vi "Highlight Selected Grey.vi"(8 "error in (no error)":errorcluster, 10 "Grey Scale Index (0-255)":u8, 11 "ColorSelector in":refnum<class "ColorSelector.lvclass">) -> (0 "error out":errorcluster, 3 "ColorSelector (dup)":refnum<class "ColorSelector.lvclass">)   [LabVIEW 2015, in "ColorSelector.lvclass"]
doc: "This VI draws the crosshairs on the correct coordinate in the Grey Selector.\n<b> </b> <b> </b>\n©2017 Q Software Innovations, LLC (QSI)\nwritten by Quentin Alldredge\nproduced in LabVIEW 2015\n\nsupport@qsoftwareinnovations.com\nwww.qsoftwareinnovations.com\n\nAll rights reserved.\n\nRedistribution and use in source and binary forms, with or without modification, are permitted provided that the following conditions are met:\n\n * Redistributions of source code must retain the above copyright notice, this list of conditions and the following disclaimer.\n * Redistributions in binary form must reproduce the above copyright notice, this list of conditions and the following disclaimer in the documentation and/or other materials provided with the distribution.\n * Neither the name of Q Software Innovations, LLC. nor the names of its contributors may be used to endorse or promote products derived from this software without specific prior written permission.\n\nTHIS SOFTWARE IS PROVIDED BY THE COPYRIGHT HOLDERS AND CONTRIBUTORS \"AS IS\" AND ANY EXPRESS OR IMPLIED WARRANTIES, INCLUDING, BUT NOT LIMITED TO, THE IMPLIED WARRANTIES OF MERCHANTABILITY AND FITNESS FOR A PARTICULAR PURPOSE ARE DISCLAIMED. IN NO EVENT SHALL THE COPYRIGHT OWNER OR CONTRIBUTORS BE LIABLE FOR ANY DIRECT, INDIRECT, INCIDENTAL, SPECIAL, EXEMPLARY, OR CONSEQUENTIAL DAMAGES (INCLUDING, BUT NOT LIMITED TO, PROCUREMENT OF SUBSTITUTE GOODS OR SERVICES; LOSS OF USE, DATA, OR PROFITS; OR BUSINESS INTERRUPTION) HOWEVER CAUSED AND ON ANY THEORY OF LIABILITY, WHETHER IN CONTRACT, STRICT LIABILITY, OR TORT (INCLUDING NEGLIGENCE OR OTHERWISE) ARISING IN ANY WAY OUT OF THE USE OF THIS SOFTWARE, EVEN IF ADVISED OF THE POSSIBILITY OF SUCH DAMAGE."
uses:
  ColorSelector.lvclass
  ColorSelector.lvclass/ColorSelector.ctl
  Read GreySelectPic.vi
  Read GreyGridCoords.vi
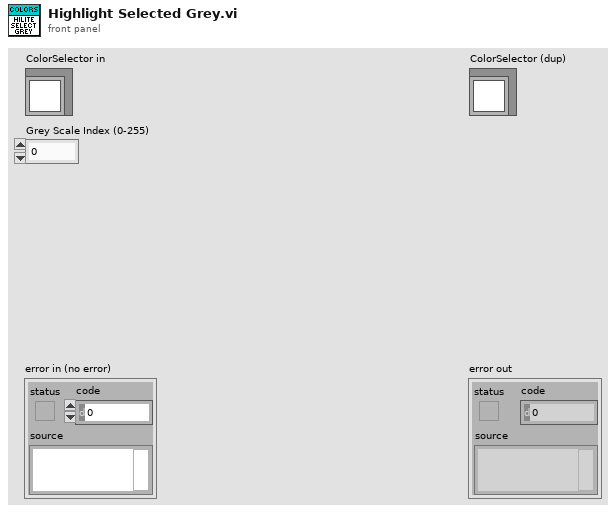
[diagram p1: front panel]
types:
  T1 = cluster{"Width":i16, "Style":enum32{"Solid", "Dash", "Dot", "DashDot", "DashDotDot"}}
  T2 = cluster{"left":i16, "top":i16, "right":i16, "bottom":i16}
  T3 = typedef "LVPoint32TypeDef.ctl" = cluster{"Horizontal":i32, "Vertical":i32}
  T4 = typedef "imagedata.ctl" = cluster{"image type":i32, "image depth":i32, "image":u8[], "mask":u8[], "colors":u32[], "Rectangle":cluster{"left":i16, "top":i16, "right":i16, "bottom":i16}}
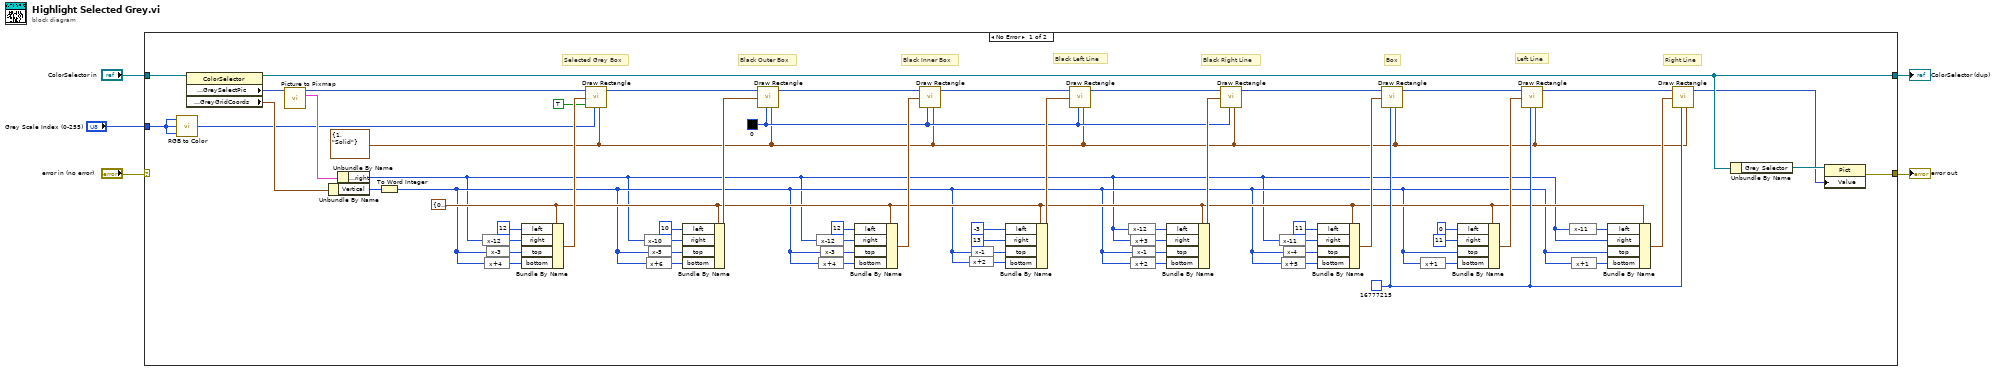
[diagram p0: block diagram]
diagram:
  n1 = case shown="No Error" "error in (no error)" {
    selector: "error in (no error)" -> [_ w70]
    tunnel: [w56 w70] -> w4
    tunnel: [w61 w69] -> w2
    tunnel: "ColorSelector in" -> [w68 w69]
    tunnel: "Grey Scale Index (0-255)" -> [w11 _]
    frame No Error {
      w31 = u32 16777215 ("color(black)")
      w23 = u32 0 ("color(black)")
      w10 = T1 {"Width"=1, "Style"=enum."Solid"} ("pen")
      w9 = T2 {"left"=0, "top"=0, "right"=0, "bottom"=0} ("rect")
      # "Selected Grey Box"
      # "Black Inner Box"
      # "Right Line"
      # "Left Line"
      # "Box"
      # "Black Right Line"
      # "Black Left Line"
      # "Black Outer Box"
      n2 = call <vilib>:"RGB to Color.vi"("B"=w11, "G"=w11, "R"=w11) -> ("Color"=w12:u32)
      n3 = property class="ColorSelector"(reference=w68) -> (reference out=w61:refnum<class "ColorSelector.lvclass">, "State Data:Accessors:GreySelectPic"=w67:picture, "State Data:Accessors:GreyGridCoords"=w59:T3)  [unwired: 1 in, 1 out]
      n4 = call <vilib>:"Picture to Pixmap.vi"("picture"=w67) -> ("image data"=w66:T4, "new picture"=w14:picture)  [unwired: 9 in]
      n5 = Unbundle By Name(w59) -> ("Vertical"=w58:i32)
      n6 = Unbundle By Name(w66) -> ("Rectangle.right"=w7:i16)
      n7 = To Word Integer(number=w58) -> (16bit integer=w8:i16)
      n8 = expression code="x-12"(w7) -> (w16:i16)
      n9 = expression code="x+4"(w8) -> (w18:i16)
      n10 = expression code="x-3"(w8) -> (w17:i16)
      n11 = Bundle By Name(cluster=w9, "left"=i16 12, "right"=w16, "top"=w17, "bottom"=w18) -> (w19:T2)
      n12 = call <vilib>:"Draw Rectangle.vi"("picture"=w14, "rect"=w19, "fill?(F)"=TRUE, "color(black)"=w12, "pen"=w10) -> ("new picture"=w13:picture)  [unwired: 4 in]
      n13 = expression code="x-10"(w7) -> (w39:i16)
      n14 = expression code="x+6"(w8) -> (w60:i16)
      n15 = expression code="x-5"(w8) -> (w55:i16)
      n16 = Bundle By Name(cluster=w9, "left"=i16 10, "right"=w39, "top"=w55, "bottom"=w60) -> (w65:T2)
      n17 = call <vilib>:"Draw Rectangle.vi"("picture"=w13, "rect"=w65, "color(black)"=w23, "pen"=w10) -> ("new picture"=w25:picture)  [unwired: 5 in]
      n18 = expression code="x-12"(w7) -> (w29:i16)
      n19 = expression code="x+4"(w8) -> (w27:i16)
      n20 = expression code="x-3"(w8) -> (w28:i16)
      n21 = Bundle By Name(cluster=w9, "left"=i16 12, "right"=w29, "top"=w28, "bottom"=w27) -> (w26:T2)
      n22 = call <vilib>:"Draw Rectangle.vi"("picture"=w25, "rect"=w26, "color(black)"=w23, "pen"=w10) -> ("new picture"=w24:picture)  [unwired: 5 in]
      n23 = expression code="x+2"(w8) -> (w42:i16)
      n24 = expression code="x-1"(w8) -> (w22:i16)
      n25 = Bundle By Name(cluster=w9, "left"=i16 -3, "right"=i16 13, "top"=w22, "bottom"=w42) -> (w63:T2)
      n26 = call <vilib>:"Draw Rectangle.vi"("picture"=w24, "rect"=w63, "color(black)"=w23, "pen"=w10) -> ("new picture"=w64:picture)  [unwired: 5 in]
      n27 = expression code="x-12"(w7) -> (w21:i16)
      n28 = expression code="x+3"(w7) -> (w53:i16)
      n29 = expression code="x+2"(w8) -> (w40:i16)
      n30 = expression code="x-1"(w8) -> (w20:i16)
      n31 = Bundle By Name(cluster=w9, "left"=w21, "right"=w53, "top"=w20, "bottom"=w40) -> (w62:T2)
      n32 = call <vilib>:"Draw Rectangle.vi"("picture"=w64, "rect"=w62, "color(black)"=w23, "pen"=w10) -> ("new picture"=w50:picture)  [unwired: 5 in]
      n33 = expression code="x-11"(w7) -> (w41:i16)
      n34 = expression code="x+5"(w8) -> (w47:i16)
      n35 = expression code="x-4"(w8) -> (w48:i16)
      n36 = Bundle By Name(cluster=w9, "left"=i16 11, "right"=w41, "top"=w48, "bottom"=w47) -> (w46:T2)
      n37 = call <vilib>:"Draw Rectangle.vi"("picture"=w50, "rect"=w46, "color(black)"=w31, "pen"=w10) -> ("new picture"=w51:picture)  [unwired: 5 in]
      n38 = expression code="x+1"(w8) -> (w34:i16)
      n39 = Bundle By Name(cluster=w9, "left"=i16 0, "right"=i16 11, "top"=w8, "bottom"=w34) -> (w44:T2)
      n40 = call <vilib>:"Draw Rectangle.vi"("picture"=w51, "rect"=w44, "color(black)"=w31, "pen"=w10) -> ("new picture"=w52:picture)  [unwired: 5 in]
      n41 = expression code="x-11"(w7) -> (w33:i16)
      n42 = expression code="x+1"(w8) -> (w32:i16)
      n43 = Bundle By Name(cluster=w9, "left"=w33, "right"=w7, "top"=w8, "bottom"=w32) -> (w43:T2)
      n44 = call <vilib>:"Draw Rectangle.vi"("picture"=w52, "rect"=w43, "color(black)"=w31, "pen"=w10) -> ("new picture"=w49:picture)  [unwired: 5 in]
      n45 = Unbundle By Name(w61) -> ("Grey Selector"=w57:refnum<vi>)
      n46 = property on="Property Node" class="Pict"(reference=w57, "Value"=w49) -> (error out=w56:errorcluster)  [unwired: 1 in, 1 out]
    }
    frame Error {
    }
  }
  "error out" <- w4
  "ColorSelector (dup)" <- w2
